vi "Read Diode.vi"(8 "error in (no error)":errorcluster, 11 "NI DMM in":refnum<class "NI DMM.lvclass">) -> (0 "error out":errorcluster, 2 "Diode Voltage":dbl, 3 "NI DMM out":refnum<class "NI DMM.lvclass">)   [LabVIEW 2010, in "NI DMM.lvclass"]
uses:
  NI DMM.lvclass
  <instrlib>/niDMM/nidmm.llb/niDMM Current Source.ctl
  <instrlib>/niDMM/nidmm.llb/niDMM Function.ctl
  NI DMM.lvclass/NI DMM.ctl
  <instrlib>/niDMM/nidmm.llb/niDMM Configure Measurement Digits.vi
panel:
  in  "Measurement Type":T1=enum."Diode"
  in  "Current Source (Amps)":T2=0.001 items=["1uA"=1e-06, "10uA"=1e-05, "100uA"=0.0001, "1mA"=0.001]
  in  "Range (Volts)":dbl=2.0 format="%.2p"
  in  "Resolution (Digits)":dbl(ring)=5.5 items=["3 1/2"=3.5, "4 1/2"=4.5, "5 1/2"=5.5, "6 1/2"=6.5, "7 1/2"=7.5]
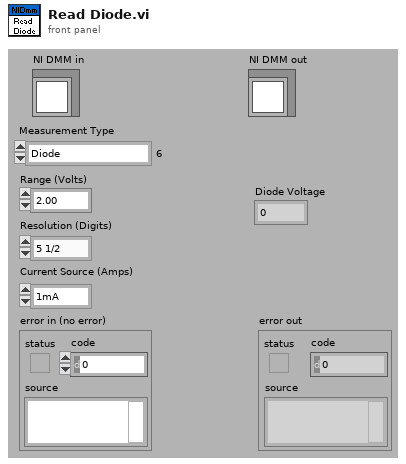
[diagram p1: front panel]
types:
  T1 = typedef "niDMM Function.ctl" = enum16{"DC Volts", "AC Volts", "DC Current", "AC Current", "2-wire Resistance", "4-wire Resistance", "Diode", "Frequency", "Period", "AC Volts DC Coupled", "Capacitance", "Inductance", "Temperature"}
  T2 = typedef "niDMM Current Source.ctl" = dbl
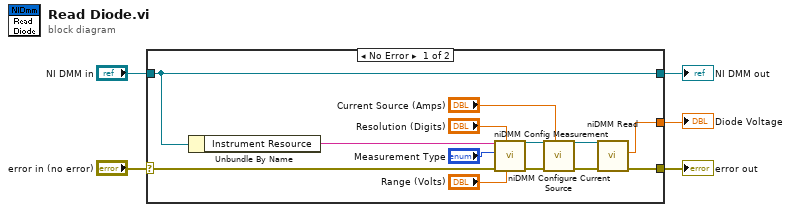
[diagram p0: block diagram]
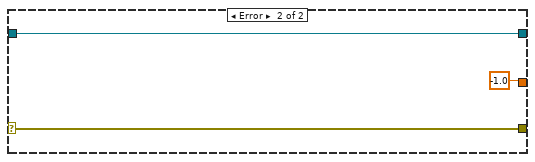
[diagram p2: hidden frame]
diagram:
  n1 = case shown="No Error" "error in (no error)" {
    selector: "error in (no error)" -> [w8 w21]
    tunnel: [w10 w21] -> w4
    tunnel: [w9 -1.0 ("Reading")] -> w3
    tunnel: "NI DMM in" -> [w7 w19]
    tunnel: [w7 w19] -> w1
    frame No Error {
      n2 = Unbundle By Name(w7) -> ("Instrument Resource"=w6:string)
      n3 = call-poly <instrlib>:"niDMM Config Measurement.vi"("Range"="Range (Volts)", "Resolution in Digits"="Resolution (Digits)", "error in (no error)"=w8, "Function"="Measurement Type", "instrument handle"=w6) -> ("error out"=w11:errorcluster, "instrument handle out"=w12:refnum<k15>)  [unwired: 5 out]
      n4 = call <instrlib>:"niDMM Configure Current Source.vi"("Current Source"="Current Source (Amps)", "error in (no error)"=w11, "instrument handle"=w12) -> ("error out"=w14:errorcluster, "instrument handle out"=w13:refnum<k15>)  [unwired: 1 in, 6 out]
      n5 = call <instrlib>:"niDMM Read.vi"("error in (no error)"=w14, "instrument handle"=w13) -> ("error out"=w10:errorcluster, "Measurement"=w9:dbl)  [unwired: 1 in, 7 out]
    }
    frame Error {
    }
  }
  "error out" <- w4
  "NI DMM out" <- w1
  "Diode Voltage" <- w3
